vi "WPI_DashboardUpdate RPC Info.vi"(11 "Operation":enum16{"Update", "Clear"}(ring)=enum."Clear") -> (2 "update":bool, 3 "commands":string[][](array[string]))   [LabVIEW 2017]
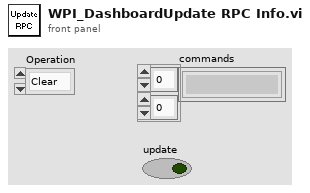
[diagram p1: front panel]
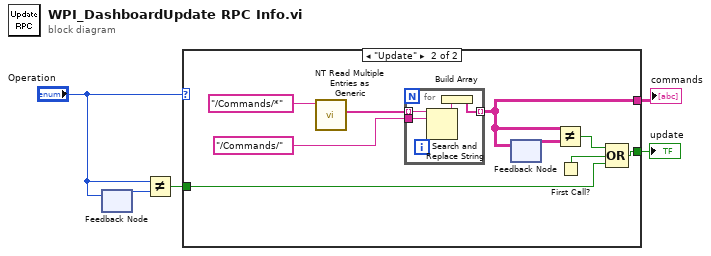
[diagram p0: block diagram]
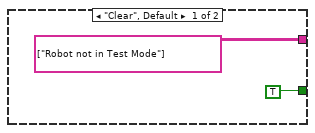
[diagram p2: hidden frame]
diagram:
  n1 = feedback #1() -> (w3:enum16{"Update", "Clear"})  [unwired: 1 in]
  n2 = feedback-in #1("Operation") -> ()
  n3 = Not Equal?(x="Operation", y=w3) -> (x != y?=w1:bool)
  n4 = case shown="\"Update\"" "Operation" {
    tunnel: [TRUE w14] -> w5
    tunnel: [string[][] [["Robot not in Test Mode"]] w13] -> w4
    tunnel: w1 -> [_ w8]
    frame "Clear", Default {
    }
    frame "Update" {
      n5 = call <vilib>:"NT Read Multiple Entries as Generic.vi"("Name Pattern"="/Commands/*") -> ("Names"=w11:string[])  [unwired: 8 in, 2 out]
      n6 = for {
        tunnel: w11 -> [w20] mode=indexing
        tunnel: "/Commands/" ("Name Pattern") -> [w19]
        tunnel: [w17] -> w13 mode=indexing
        n7 = Search and Replace String(input string=w20, search string=w19) -> (result string=w18:string)  [unwired: 6 in, 3 out]
        n8 = Build Array(w18) -> (w17:string[])
      }
      n9 = feedback #2() -> (w12:string[][])  [unwired: 1 in]
      n10 = feedback-in #2(w13) -> ()
      n11 = Not Equal?(x=w13, y=w12) -> (x != y?=w15:bool)
      n12 = First Call?() -> (First Call?: T/F=w16:bool)
      n13 = Compound Arithmetic op=OR(w15, w16, w8) -> (w14:bool)
    }
  }
  "update" <- w5
  "commands" <- w4
